vi "unpack_rm_vlc.vi"(11 "payload":u64) -> (1 "error":bool, 2 "rm_vlc_metadata":T1, 3 "image":u8[][](array[numeric]))   [LabVIEW 2023]
panel:
  in  "rm_vlc_metadata":T1
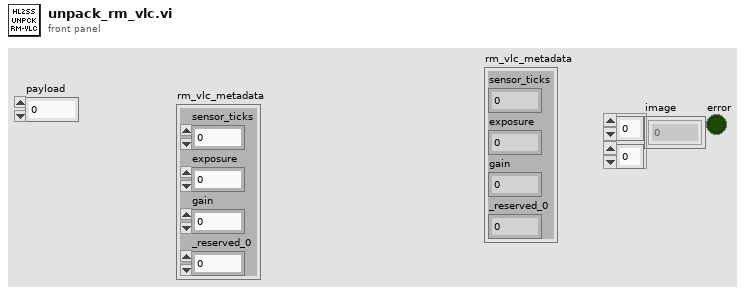
[diagram p1: front panel]
types:
  T1 = cluster{"sensor_ticks":u64, "exposure":u64, "gain":u32, "_reserved_0":u32}
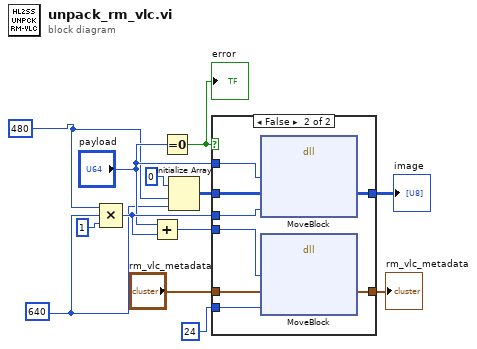
[diagram p0: block diagram]
diagram:
  w2 = u16 640 ("value")
  w3 = u16 480 ("value")
  n1 = Compound Arithmetic op=MULTIPLY(w3, w2, u64 1 ("value")) -> (w10:u64)
  n2 = Add(x="payload", y=w10) -> (x+y=w9:u64)
  n3 = Equal To 0?(x="payload") -> (x = 0?=w4:bool)
  "error" <- w4
  n4 = Initialize Array(u8 0, w3, w2) -> (w11:u8[][])
  n5 = case shown="False" w4 {
    tunnel: w11 -> [w15 w23]
    tunnel: "payload" -> [_ w22]
    tunnel: w10 -> [_ w21]
    tunnel: w9 -> [_ w20]
    tunnel: u64 24 ("size") -> [_ w19]
    tunnel: "rm_vlc_metadata" -> [w14 w18]
    tunnel: [w15 w17] -> w6
    tunnel: [w14 w16] -> w1
    frame True {
    }
    frame False {
      n6 = dll-call lib="LabVIEW" fn="MoveBlock"("ps"=w22, "pd"=w23, "size"=w21) -> ("pd"=w17:u8[][])  [unwired: 6 in, 2 out]
      n7 = dll-call lib="LabVIEW" fn="MoveBlock"("ps"=w20, "pd"=w18, "size"=w19) -> ("pd"=w16:T1)  [unwired: 6 in, 2 out]
    }
  }
  "image" <- w6
  "rm_vlc_metadata" <- w1
